vi "host.bats.parser.tester.vi"() -> ()   [LabVIEW 2020]
uses:
  arty/orderbook/orderbook.command.data.ctl
  arty/orderbook/orderbook.command.type.ctl
  <vilib>/rvi/interface/RandomDataEmulation/nirviRandomDataOpen.vi
  <vilib>/rvi/interface/common/niFpgaCacheSessionInfoDynamic.vi
  <vilib>/Utility/error.llb/Error Cluster From Error Code.vi
  <vilib>/rvi/errors/niLvFpgaAdjustHostInterfaceError.vi
  <vilib>/FPGAPlugInAG/Dynamic/niLvFpga_Close_Dynamic.vi
  <vilib>/rvi/interface/nirviOpenFPGA/nirviOpenFPGA.xnode
  arty/bats.parser/fpga.bats.parser.test.harness.vi
  <vilib>/rvi/interface/nirviReadWriteControl/nirviReadWriteControl.xnode
  <vilib>/rvi/interface/nirviMethod/nirviMethod.xnode
  <vilib>/rvi/interface/nirviCloseFPGA/nirviCloseFPGA.xnode
  <vilib>/rvi/errors/niLvFpgaMergeErrorWithErrorCode.vi
  <vilib>/FPGAPlugInAG/Dynamic/niLvFpga_ReadFifo_Dynamic.vi
  NiFpgaLv.dll
  <vilib>/rvi/interface/Simulation/niFpgaSimulationCallBeginRW.vi
  <vilib>/FPGAPlugInAG/Dynamic/niLvFpga_WriteFifo_Dynamic.vi
panel:
  in  "Trim Input\nData?":bool=TRUE
  in  "# of elements\n to send":i32=50
  out "OrderBook.Command[]":T1[](array[typedef]) {"Side (U8)" format="%.0x"; "Order Id (U64)" format="%.0x"; "Symbol (U64)" format="%.0x"}
  out "Data.size":i32=8
  out "DataToSend.size":i32
  in  "Execute?":bool=TRUE
  in  "BATS Data File":string="raw.pitch.dat"
  out "Data":u64[](array[numeric]) format="%.0x"
  out "error out":errorcluster
  in  "error in":errorcluster
  out "DataToSend":u16[](array[numeric]) format="%.0x"
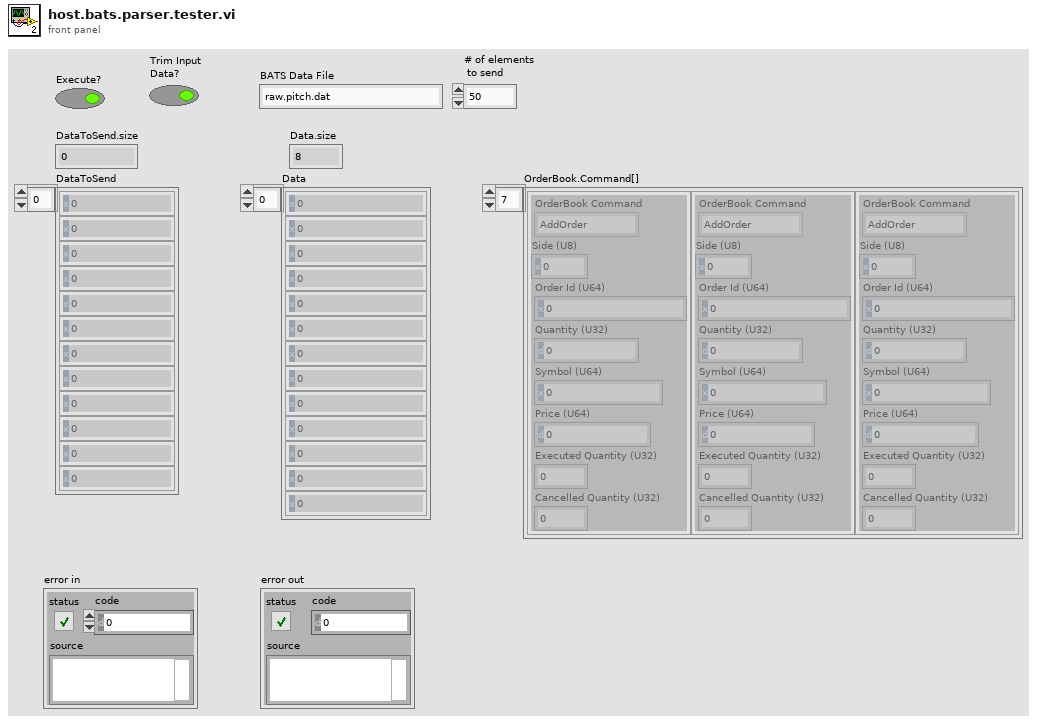
[diagram p1: front panel]
types:
  T1 = typedef "orderbook.command.data.ctl" = cluster{"OrderBook Command":T2, "Side (U8)":u8, "Order Id (U64)":u64, "Quantity (U32)":u32, "Symbol (U64)":u64, "Price (U64)":u64, "Executed Quantity (U32)":u32, "Cancelled Quantity (U32)":u32}
  T2 = typedef "orderbook.command.type.ctl" = enum16{"AddOrder", "OrderExecuted", "ReduceSize", "ModifyOrder", "DeleteOrder"}
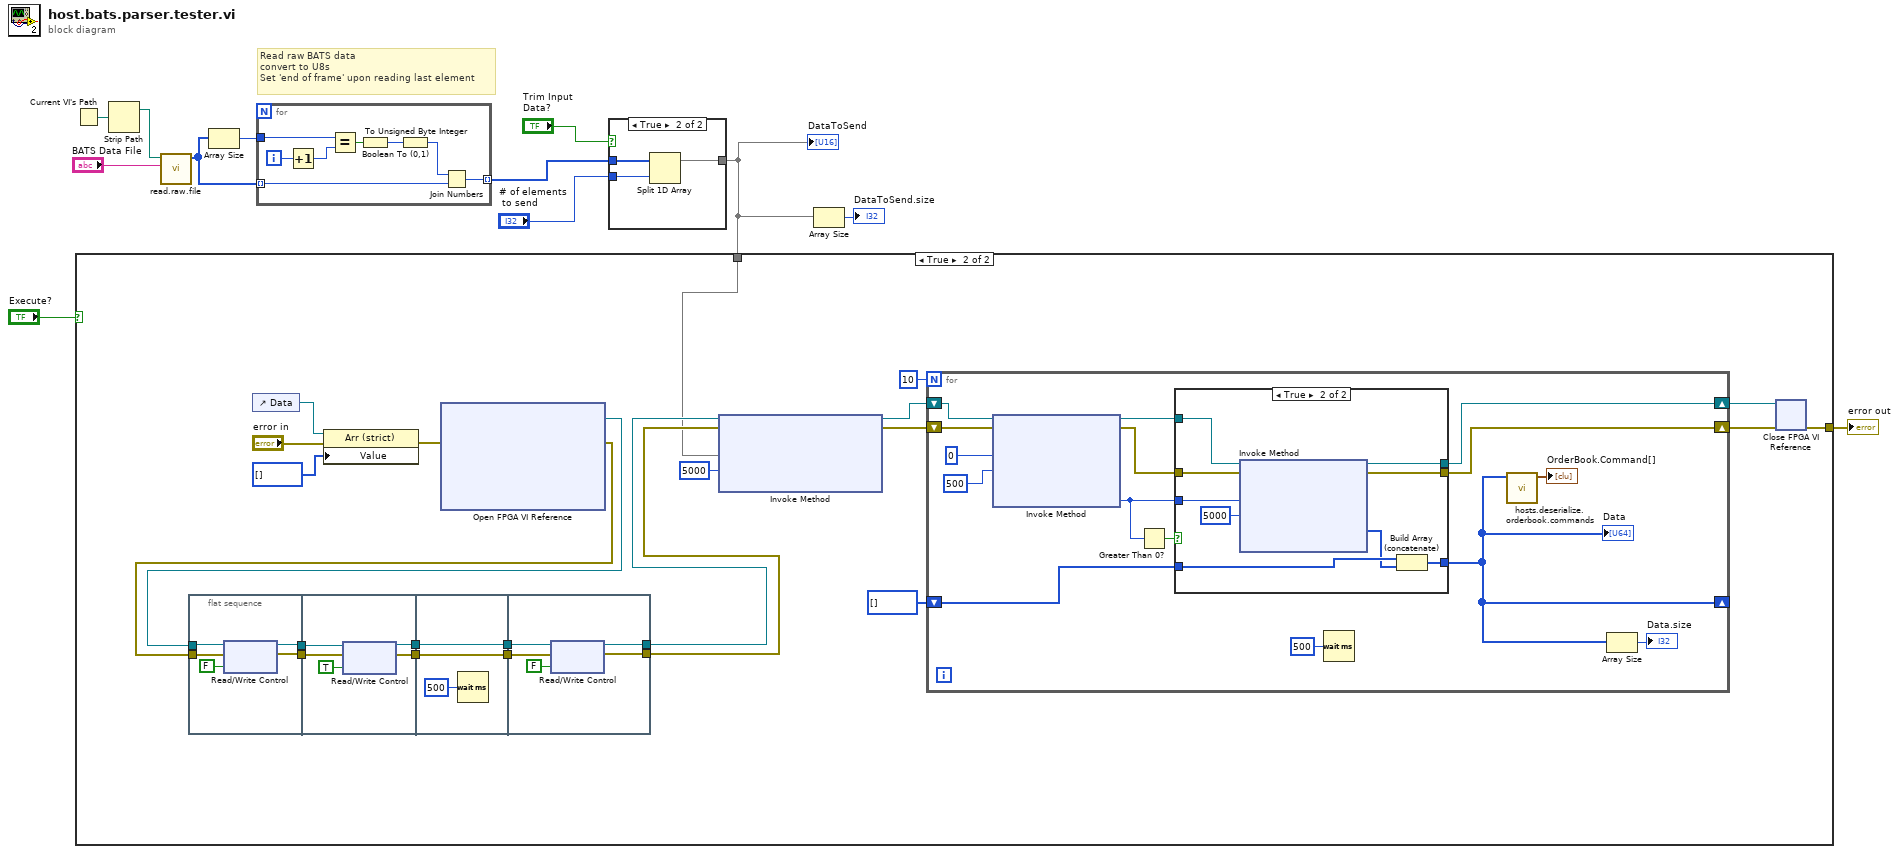
[diagram p0: block diagram]
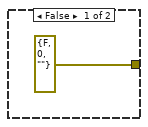
[diagram p3: hidden frame]
diagram:
  # "Read raw BATS data\nconvert to U8s\nSet 'end of frame' upon reading last element"
  n1 = Current VI's Path() -> (path=w10:path)
  n2 = Strip Path(path=w10) -> (stripped path=w8:path)  [unwired: 1 out]
  n3 = call "read.raw.file.vi"("Raw File"="BATS Data File", "Path"=w8) -> ("data"=w7:u8[])  [unwired: 9 in]
  n4 = Array Size(array=w7) -> (size(s)=w12:i32)
  n5 = for {
    tunnel: w7 -> [w18] mode=indexing
    tunnel: w12 -> [w20]
    tunnel: [w14] -> w4 mode=indexing
    i -> [w19]
    n6 = Increment(x=w19) -> (x+1=w13:i32)
    n7 = Equal?(x=w20, y=w13) -> (x = y?=w17:bool)
    n8 = Boolean To (0,1)(Boolean=w17) -> (0, 1=w16:i16)
    n9 = To Unsigned Byte Integer(number=w16) -> (unsigned 8bit integer=w15:u8)
    n10 = Join Numbers(hi=w15, lo=w18) -> ((hi.lo)=w14:u16)
  }
  n11 = case shown="True" "Trim Input\nData?" {
    tunnel: w4 -> [w21 w24]
    tunnel: "# of elements\n to send" -> [_ w23]
    tunnel: [w21 w22] -> w2
    frame False {
    }
    frame True {
      n12 = Split 1D Array(array=w24, index=w23) -> (first subarray=w22:u16[])  [unwired: 1 out]
    }
  }
  "DataToSend" <- w2
  n13 = case shown="True" "Execute?" {
    tunnel: [errorcluster {"status"=FALSE, "code"=0, "source"=""} ("error out") w48] -> w11
    tunnel: w2 -> [_ w30]
    frame False {
    }
    frame True {
      n14 = flat-sequence {
        tunnel: w31 -> [w50]
        tunnel: w32 -> [w51]
        tunnel: [w52] -> w29
        tunnel: [w53] -> w28
        tunnel: [w57] -> w37
        tunnel: [w56] -> w36
        tunnel: w29 -> [w55]
        tunnel: w28 -> [w54]
        tunnel: [w61] -> w38
        tunnel: w37 -> [w61]
        tunnel: w36 -> [w60]
        tunnel: [w60] -> w35
        tunnel: w38 -> [w65]
        tunnel: w35 -> [w64]
        tunnel: [w63] -> w34
        tunnel: [w62] -> w33
        frame #0 {
          n15 = xnode "Read/Write Control"("FPGA VI Reference In"=w50, "error in"=w51, "reset"=FALSE) -> ("FPGA VI Reference Out"=w53:refnum<k20>, "error out"=w52:errorcluster)
        }
        frame #1 {
          n16 = xnode "Read/Write Control"("FPGA VI Reference In"=w54, "error in"=w55, "reset"=TRUE) -> ("FPGA VI Reference Out"=w56:refnum<k20>, "error out"=w57:errorcluster)
        }
        frame #2 {
          n17 = Wait (ms)(milliseconds to wait=u32 500) -> ()  [unwired: 1 out]
        }
        frame #3 {
          n18 = xnode "Read/Write Control"("FPGA VI Reference In"=w64, "error in"=w65, "reset"=FALSE) -> ("FPGA VI Reference Out"=w62:refnum<k20>, "error out"=w63:errorcluster)
        }
      }
      n19 = control-ref of="Data"() -> (w42:refnum<vi>)
      n20 = property class="Arr (strict)"(reference=w42, error in="error in", "Value"=u8[] []) -> (error out=w39:errorcluster)  [unwired: 1 out]
      n21 = xnode "Open FPGA VI Reference"("error in"=w39) -> ("FPGA VI Reference Out"=w31:refnum<k20>, "error out"=w32:errorcluster)  [unwired: 1 in]
      n22 = xnode "Invoke Method"("FPGA VI Reference In"=w33, "error in"=w34, "Data"=w30, "Timeout (ms)"=5000) -> ("FPGA VI Reference Out"=w47:refnum<k20>, "error out"=w46:errorcluster)  [unwired: 1 out]
      n23 = for {
        N: 10 -> [_]
        shift-right: [w69] -> _
        shift-left: u64[] [] -> [w74]
        shift-right: [w73] -> w44
        shift-left: w47 -> [w81]
        shift-right: [w72] -> w43
        shift-left: w46 -> [w80]
        n24 = xnode "Invoke Method"("FPGA VI Reference In"=w81, "error in"=w80, "Number of Elements"=u32 0, "Timeout (ms)"=500) -> ("FPGA VI Reference Out"=w75:refnum<k20>, "error out"=w71:errorcluster, "Elements Remaining"=w76:u32)  [unwired: 1 out]
        n25 = Greater Than 0?(x=w76) -> (x > 0?=w77:bool)
        n26 = case shown="True" w77 {
          tunnel: w76 -> [_ w93]
          tunnel: w75 -> [w83 w91]
          tunnel: [w84 w88] -> w69
          tunnel: w74 -> [w84 w90]
          tunnel: [w83 w87] -> w73
          tunnel: [w82 w86] -> w72
          tunnel: w71 -> [w82 w85]
          frame False {
          }
          frame True {
            n27 = xnode "Invoke Method"("FPGA VI Reference In"=w91, "error in"=w85, "Number of Elements"=w93, "Timeout (ms)"=5000) -> ("FPGA VI Reference Out"=w87:refnum<k20>, "error out"=w86:errorcluster, "Data"=w89:u64[])  [unwired: 1 out]
            n28 = Build Array (concatenate)(w90, w89) -> (w88:u64[])
          }
        }
        "Data" <- w69
        n29 = Wait (ms)(milliseconds to wait=u32 500) -> ()  [unwired: 1 out]
        n30 = call "hosts.deserialize.orderbook.commands.vi"("DataIn"=w69) -> ("OrderBook.Command[]"=→"OrderBook.Command[]":T1[])  [unwired: 10 in]
        n31 = Array Size(array=w69) -> (size(s)=→"Data.size":i32)
      }
      n32 = xnode "Close FPGA VI Reference"("FPGA VI Reference In"=w44, "error in"=w43) -> ("error out"=w48:errorcluster)
    }
  }
  "error out" <- w11
  n33 = Array Size(array=w2) -> (size(s)=→"DataToSend.size":i32)
